vi "main-顶层容器-网络客户端.vi"() -> ()   [LabVIEW 2017]
uses:
  21b310b3-65e2-4238-aede-b4c1b8493430.vi
panel:
  out "错误输出":errorcluster
  in  "信号-设置":bool=TRUE
  in  "子面板模式":T1
  out "浏览-刷新信号 按钮":refnum<vi>
  out "浏览-停止信号 按钮":refnum<vi>
  out "查询窗口VI-引用":refnum<vi>
  out "管-监测模式状态？":refnum<vi>
  out "管-停止信号（枚举）":refnum<vi>
  out "管-监测窗口 按钮":refnum<vi>
  in  "监-外部停止信号":refnum<vi>
  out "管理窗口VI-引用":refnum<vi>
  out "管-监测窗口VI-控件引用":refnum<vi>
  in  "管理模式":bool
  in  "监测模式":bool
  in  "浏览模式":bool
  in  "设置":bool
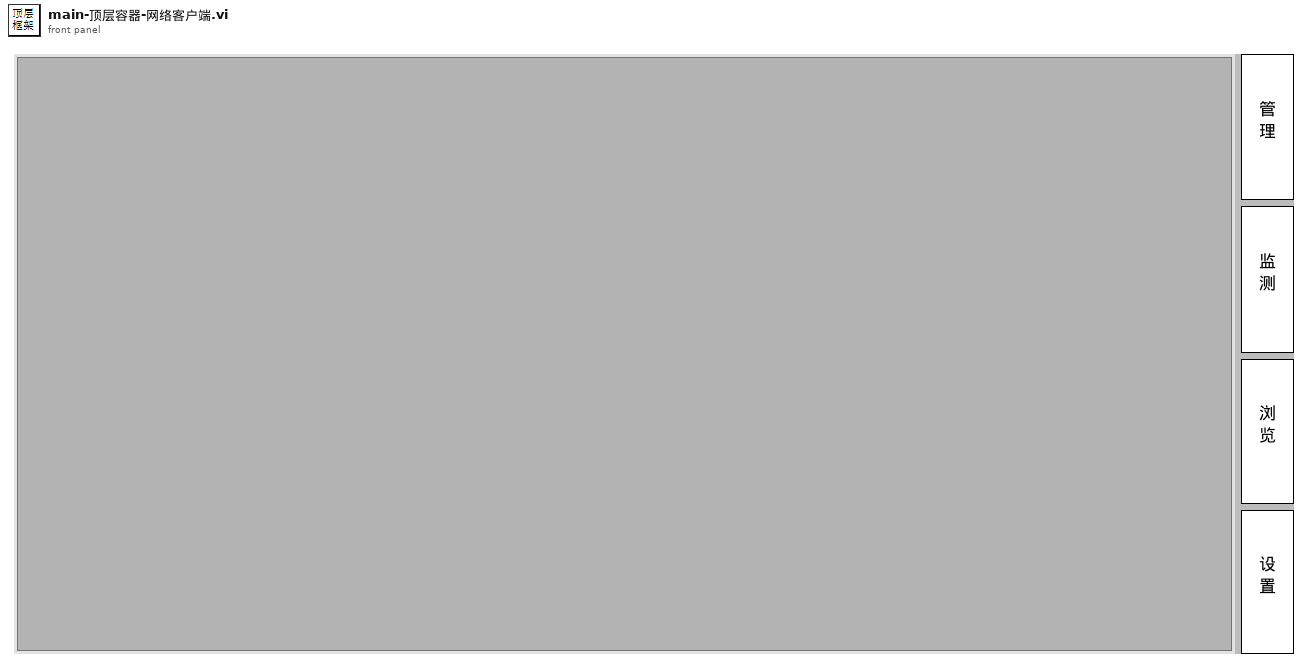
[diagram p1: front panel]
types:
  T1 = typedef "枚举-顶层框架功能模式.ctl" = enum16{"管理模式", "监测模式", "浏览模式"}
  T2 = typedef "簇-输入.ctl" = cluster{"配置文件动作":T3, "数据输入":variant}
  T3 = typedef "枚举-配置文件动作.ctl" = enum16{"初始化加载配置", "读取配置", "写入-屏幕键盘", "写入-静音延迟", "写入-主要探头类型", "写入-串口配置", "写入-累积定时", "写入-导出定时", "保存配置到文件"}
  T4 = enum8{"Enabled", "Disabled", "Disabled and Grayed Out"}
  T5 = typedef "簇-配置文件内容.ctl" = cluster{"调试模式？":bool, "屏幕键盘？":bool, "软件版本":string, "静音延迟 s":u16, "主要探头类型":T6, "串口配置":cluster{"COM口":refnum<visa-resource-name>, "波特率":enum16{"9600", "19200"}, "读写超时ms":i16, "丢包判定次数":i16}, "定时配置-累积分段":T7, "定时配置-自动导出":cluster{"定时配置-自动导出":T7, "分别导出?":bool}}
  T6 = typedef "枚举-主要探头类型.ctl" = enum16{"网络探头", "串口探头"}
  T7 = typedef "簇-定时配置.ctl" = cluster{"定时模式":enum16{"绝对时间", "相对时间"}, "单位":enum16{"年", "月", "日", "时", "分"}, "间隔":u8, "目标时刻":timestamp}
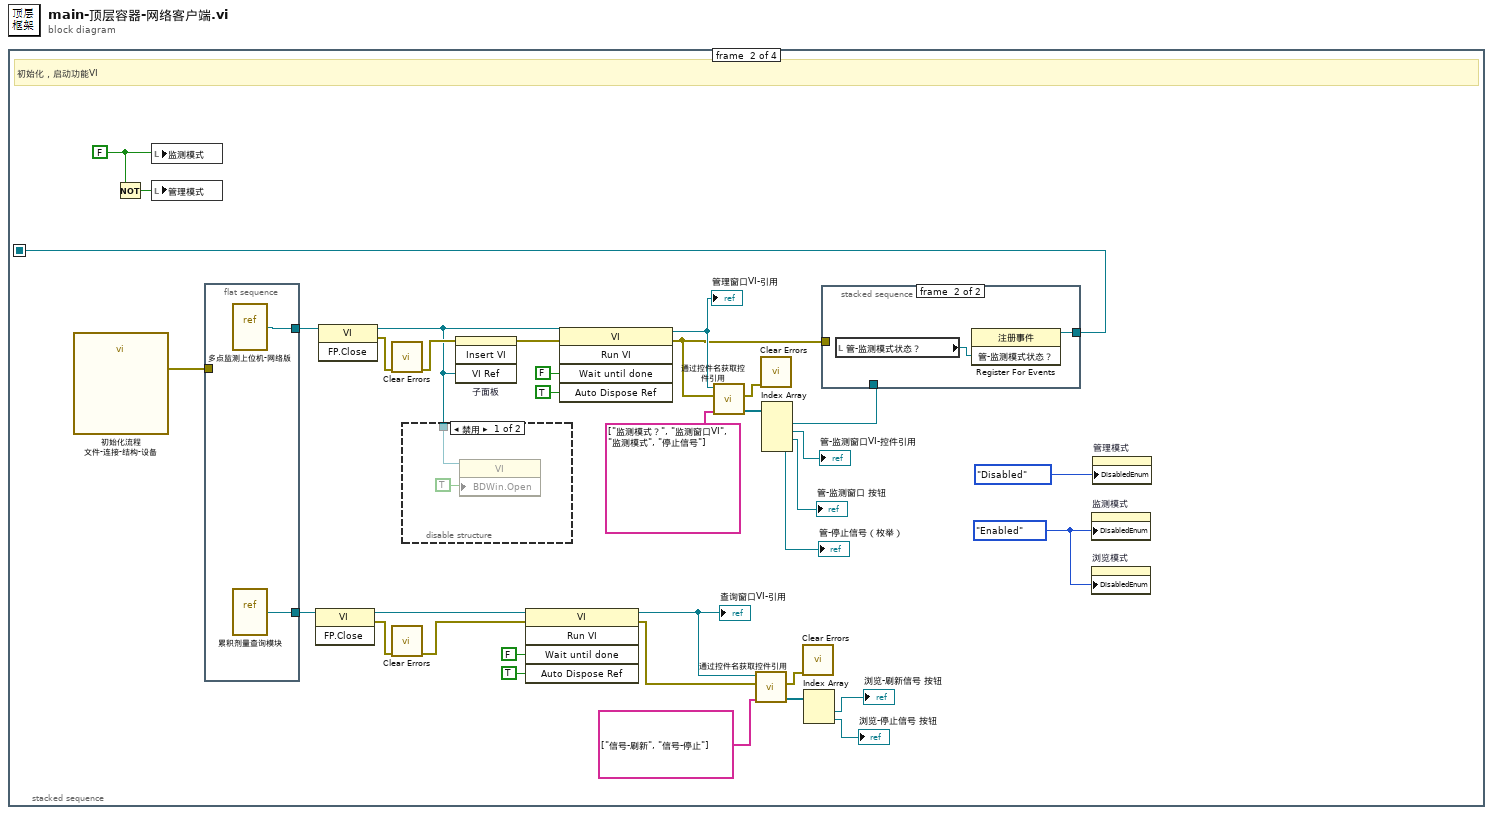
[diagram p0: block diagram]
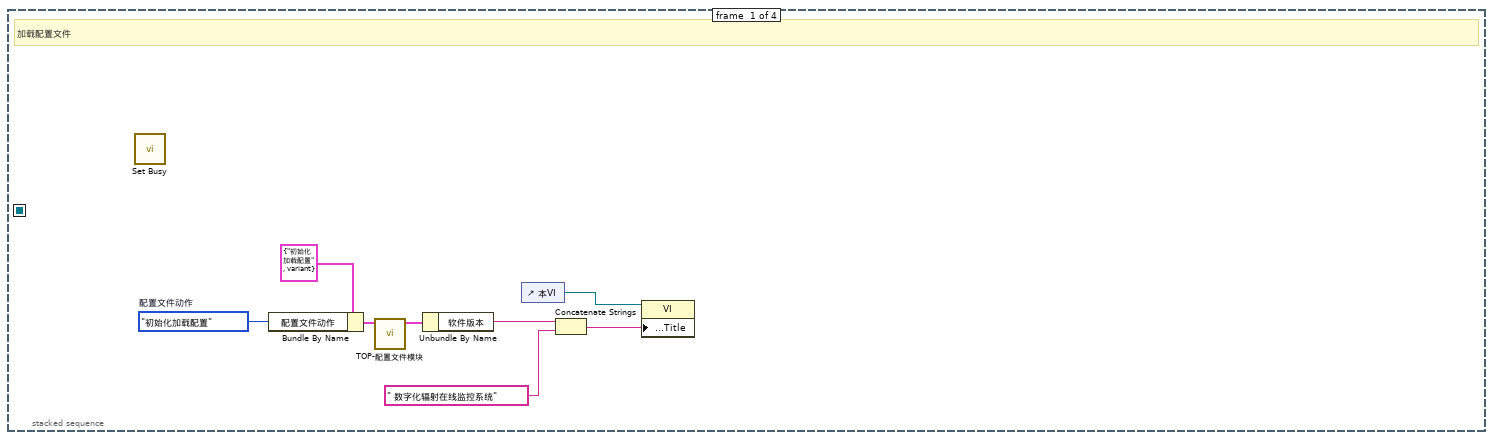
[diagram p2: hidden frame]
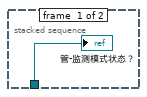
[diagram p4: hidden frame]
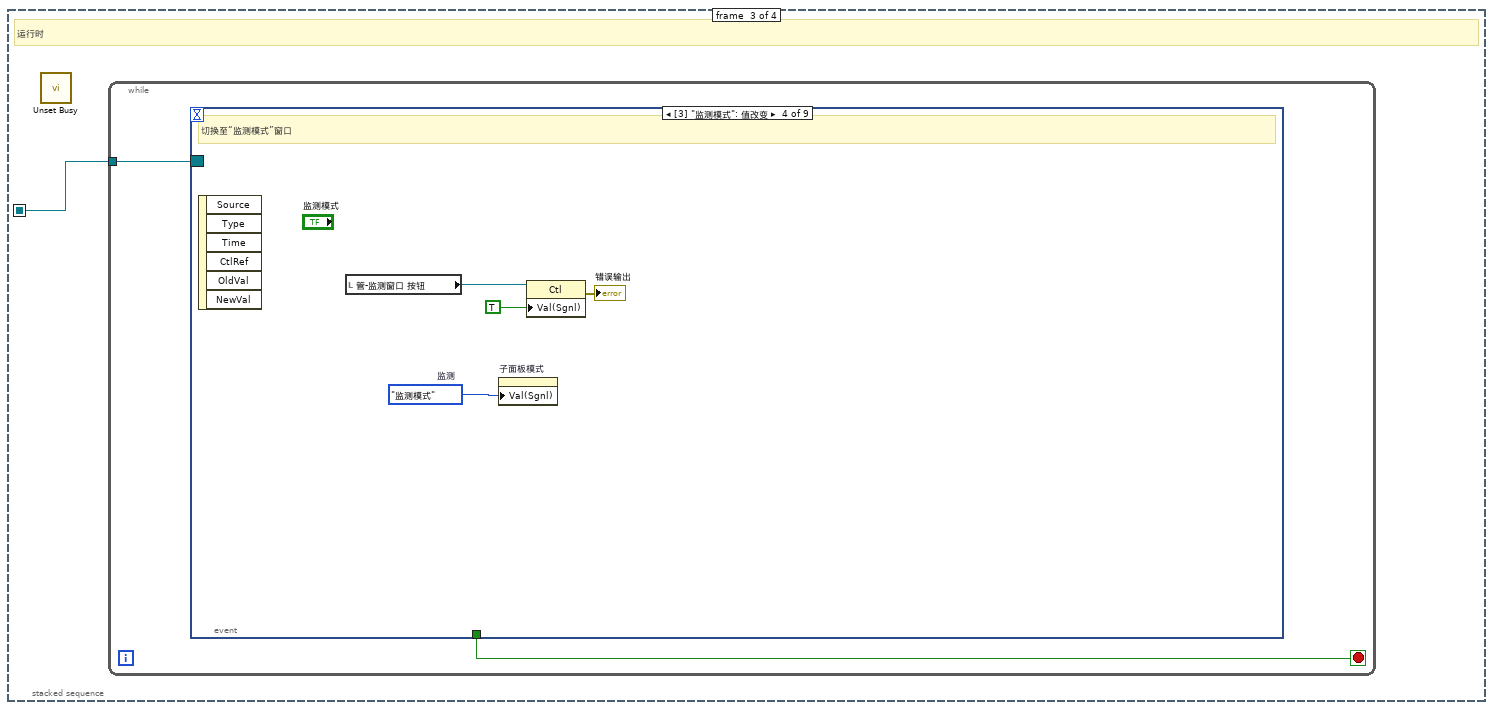
[diagram p5: hidden frame]
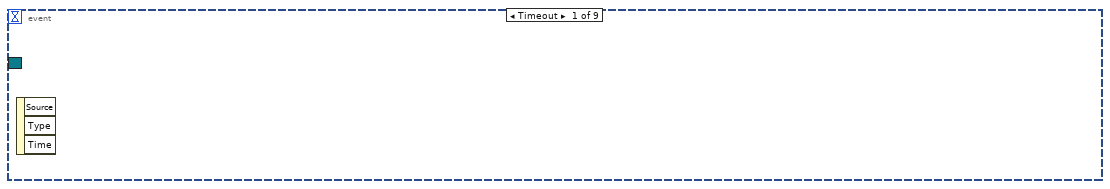
[diagram p6: hidden frame]
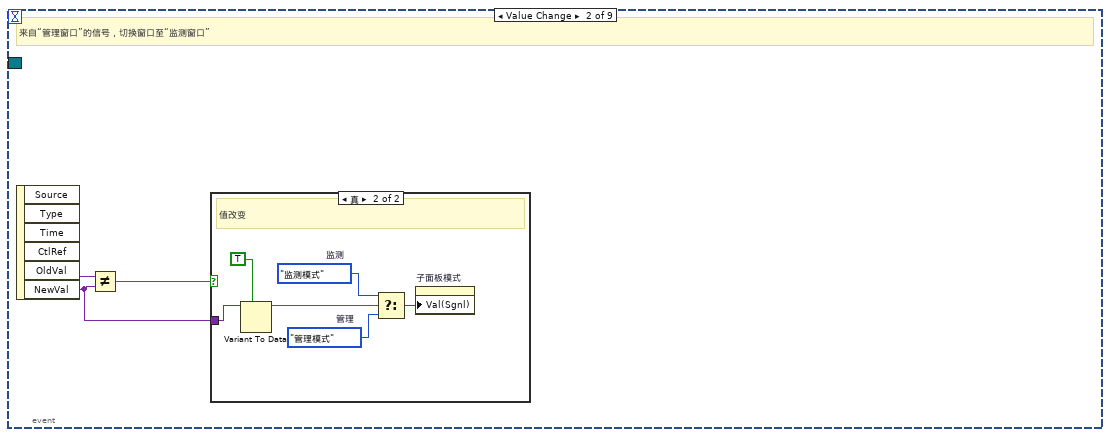
[diagram p7: hidden frame]
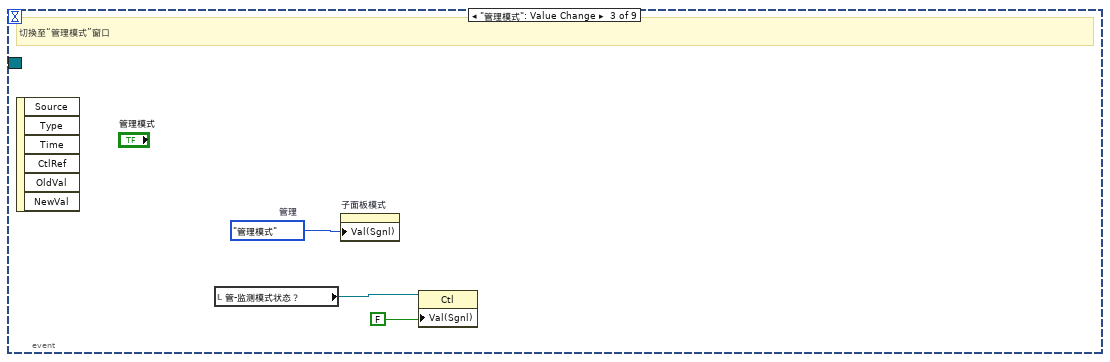
[diagram p9: hidden frame]
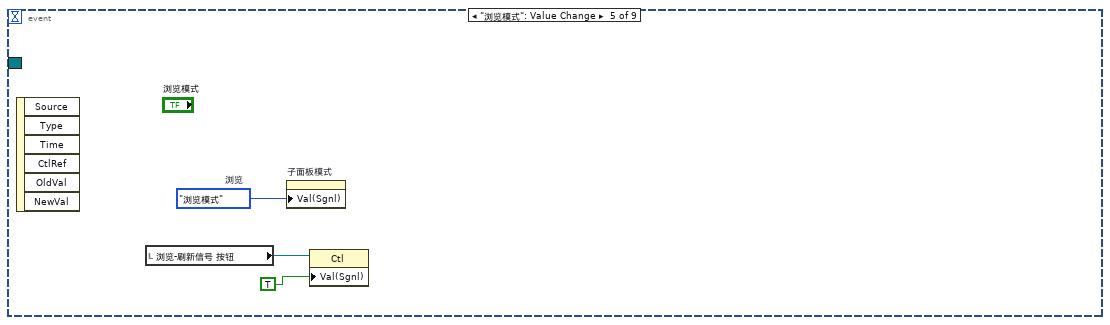
[diagram p10: hidden frame]
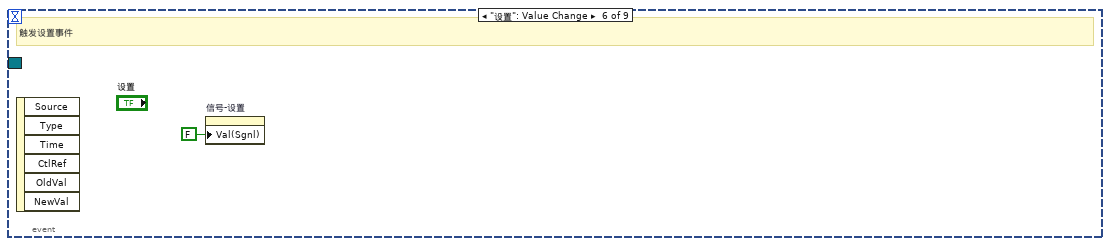
[diagram p11: hidden frame]
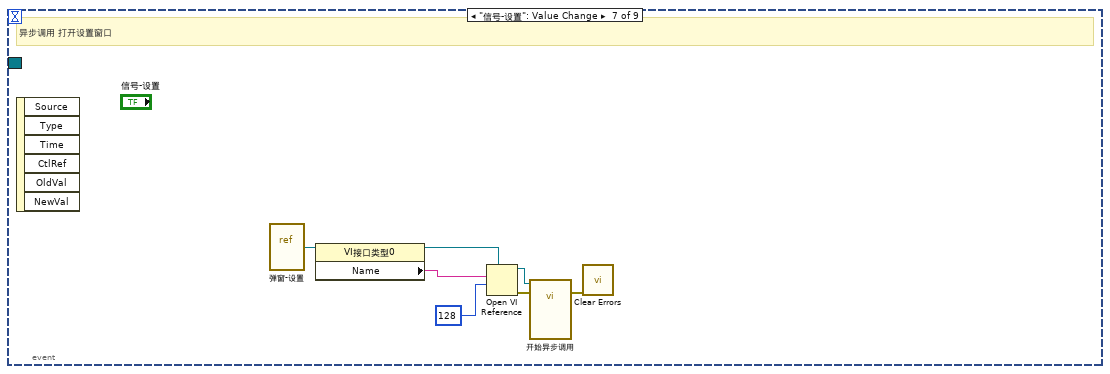
[diagram p12: hidden frame]
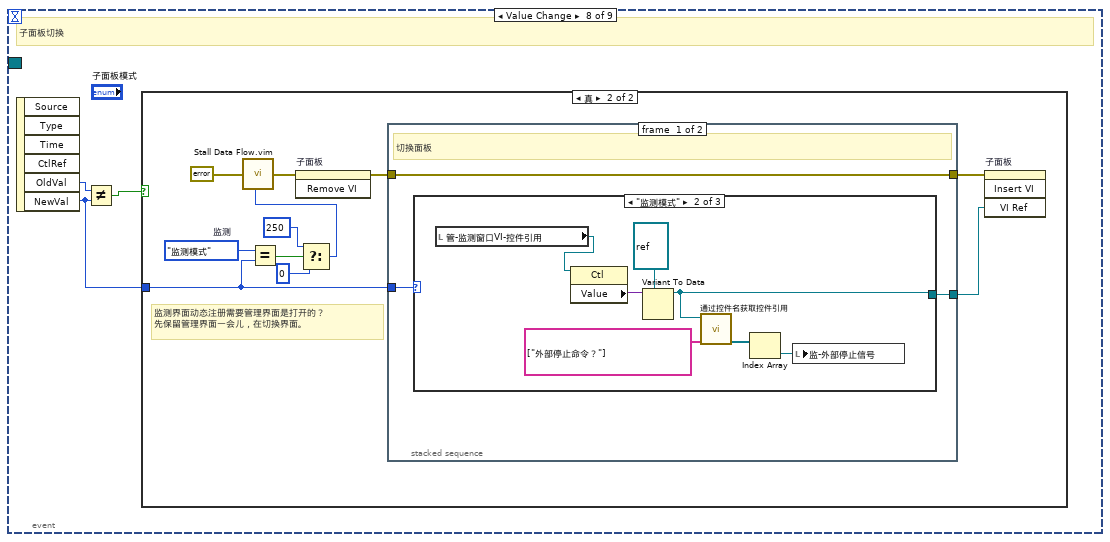
[diagram p13: hidden frame]
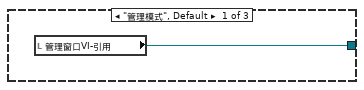
[diagram p15: hidden frame]
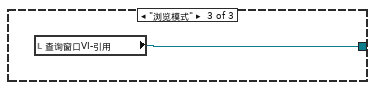
[diagram p16: hidden frame]
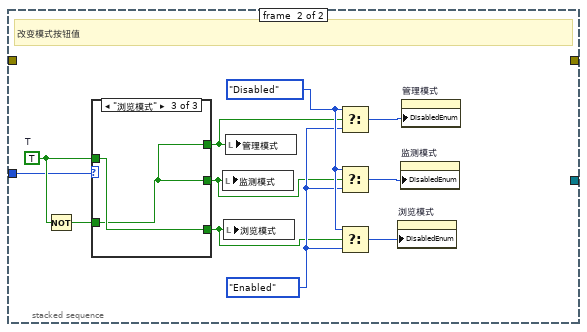
[diagram p17: hidden frame]
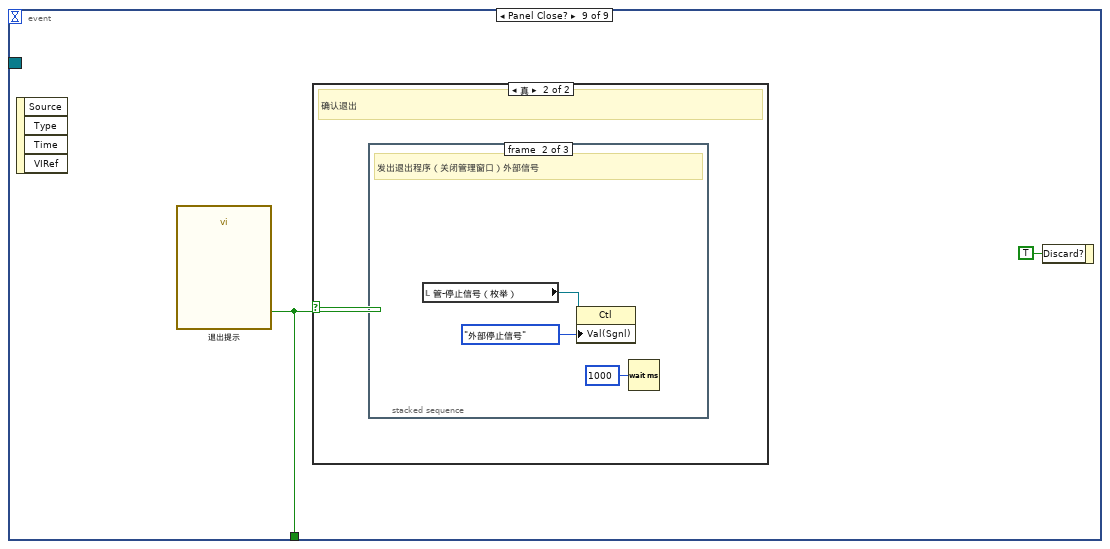
[diagram p20: hidden frame]
diagram:
  n1 = stacked-sequence {
    seq-local: [_ w36 _ _] -> [_ _ w51 _]
    frame #0 {
      w6 = 枚举-配置文件动作."初始化加载配置"  # 配置文件动作
      # "加载配置文件"
      n2 = call <vilib>:"Set Busy.vi"() -> ()  [unwired: 10 in, 2 out]
      n3 = Bundle By Name(cluster=T2 {"配置文件动作"=enum."初始化加载配置", "数据输入"=variant} ("输入"), "配置文件动作"=w6) -> (w7:T2)
      n4 = call "TOP-配置文件模块.vi"("输入"=w7) -> ("配置文件"=w5:T5)  [unwired: 9 in, 1 out]
      n5 = Unbundle By Name(w5) -> ("软件版本"=w1:string)
      n6 = control-ref of="本VI"() -> (w4:refnum<vi>)
      n7 = Concatenate Strings(w1, " 数字化辐射在线监控系统" ("前面板窗口:标题")) -> (w3:string)
      n8 = property class="VI"(reference=w4, "Front Panel.Title"=w3) -> ()  [unwired: 1 in, 2 out]
    }
    frame #1 {
      w9 = T4."Enabled" ("禁用")
      w43 = FALSE ("监测模式")
      # "初始化，启动功能VI"
      n9 = call "初始化流程 文件-连接-结构-设备.vi"() -> ("error out"=w23:errorcluster)  [unwired: 10 in, 1 out]
      n10 = Not(x=w43) -> (.not. x?=w42:bool)
      n11 = local write "监测模式"(w43) -> ()
      n12 = local write "管理模式"(w42) -> ()
      n13 = flat-sequence {
        tunnel: [w45] -> w31
        tunnel: w23 -> [_]
        tunnel: [w44] -> w21
        frame #0 {
          n14 = vi-ref "多点监测上位机-网络版.vi"() -> (w45:refnum<vi>)
          n15 = vi-ref "累积剂量查询模块.vi"() -> (w44:refnum<vi>)
        }
      }
      n16 = invoke class="VI" method="FP.Close"(reference=w21) -> (reference out=w18:refnum<vi>, error out=w22:errorcluster)  [unwired: 2 in, 1 out]
      n17 = invoke class="VI" method="FP.Close"(reference=w31) -> (reference out=w27:refnum<vi>, error out=w29:errorcluster)  [unwired: 2 in, 1 out]
      n18 = call <vilib>:"Clear Errors.vi"("error in (no error)"=w29) -> ("error out"=w28:errorcluster)  [unwired: 5 in, 1 out]
      n19 = call <vilib>:"Clear Errors.vi"("error in (no error)"=w22) -> ("error out"=w17:errorcluster)  [unwired: 5 in, 1 out]
      n20 = disable-structure shown="禁用" {
        disable-tunnel: w27 -> [w47 _]
        frame Disabled {
          n21 = property class="VI"(reference=w47, "BDWin.Open"=TRUE ("程序框图窗口:打开")) -> ()  [unwired: 1 in, 2 out]
        }
        frame Enabled {
        }
      }
      n22 = invoke on="子面板" class="子面板" method="Insert VI"(error in=w28, "VI Ref"=w27) -> (error out=w25:errorcluster)  [unwired: 2 in, 3 out]
      n23 = invoke class="VI" method="Run VI"(reference=w18, error in=w17, "Wait until done"=FALSE ("结束前等待"), "Auto Dispose Ref"=TRUE ("自动销毁引用")) -> (reference out=w13:refnum<vi>, error out=w12:errorcluster)  [unwired: 1 in, 3 out]
      "查询窗口VI-引用" <- w13
      n24 = invoke class="VI" method="Run VI"(reference=w27, error in=w25, "Wait until done"=FALSE ("结束前等待"), "Auto Dispose Ref"=TRUE ("自动销毁引用")) -> (reference out=w37:refnum<vi>, error out=w26:errorcluster)  [unwired: 1 in, 3 out]
      "管理窗口VI-引用" <- w37
      n25 = call "通过控件名获取控件引用.vi"("控件名数组"=string[] ["监测模式？", "监测窗口VI", "监测模式", "停止信号"], "错误输入（无错误）"=w26, "VI引用"=w37) -> ("控件引用输出"=w39:refnum<vi>[], "错误输出"=w30:errorcluster)  [unwired: 6 in, 1 out]
      n26 = call "通过控件名获取控件引用.vi"("控件名数组"=string[] ["信号-刷新", "信号-停止"], "错误输入（无错误）"=w12, "VI引用"=w13) -> ("控件引用输出"=w15:refnum<vi>[], "错误输出"=w16:errorcluster)  [unwired: 6 in, 1 out]
      n27 = call <vilib>:"Clear Errors.vi"("error in (no error)"=w30) -> ()  [unwired: 5 in, 2 out]
      n28 = Index Array(array=w39) -> (element #1=w24:refnum<vi>, element #2=→"管-监测窗口VI-控件引用":refnum<vi>, element #3=→"管-监测窗口 按钮":refnum<vi>, element #4=→"管-停止信号（枚举）":refnum<vi>)  [unwired: 4 in]
      n29 = call <vilib>:"Clear Errors.vi"("error in (no error)"=w16) -> ()  [unwired: 5 in, 2 out]
      n30 = Index Array(array=w15) -> (element #1=→"浏览-刷新信号 按钮":refnum<vi>, element #2=→"浏览-停止信号 按钮":refnum<vi>)  [unwired: 2 in]
      n31 = stacked-sequence {
        tunnel: [_ w50] -> w36
        tunnel: w26 -> [_ _]
        tunnel: w24 -> [w48 _]
        frame #0 {
          "管-监测模式状态？" <- w48
        }
        frame #1 {
          n32 = local read "管-监测模式状态？"() -> (w49:refnum<vi>)
          n33 = register-events(w49) -> (reference out=w50:refnum<event-registration>)  [unwired: 2 in, 1 out]
        }
      }
      n34 = property on="监测模式" class="Bool (严格)"("DisabledEnum"=w9) -> ()  [unwired: 2 in, 2 out]
      n35 = property on="浏览模式" class="Bool (严格)"("DisabledEnum"=w9) -> ()  [unwired: 2 in, 2 out]
      n36 = property on="管理模式" class="Bool (严格)"("DisabledEnum"=T4."Disabled" ("禁用")) -> ()  [unwired: 2 in, 2 out]
    }
    frame #2 {
      # "运行时"
      n37 = call <vilib>:"Unset Busy.vi"() -> ()  [unwired: 11 in, 1 out]
      n38 = while {
        tunnel: w51 -> [w52]
        stop <- w53 stop-if-true
        n39 = event shown="[3] \"监测模式\": 值改变" {
          selector: w52 -> [_ _ _ _ _ _ _ _ _]
          dyn-events: _ -> [_ _ _ _ _ _ _ _ _]
          timeout: _ -> [_ _ _ _ _ _ _ _ _]
          tunnel: [_ _ _ _ _ _ _ _ w124] -> w53
          event Timeout {
            n40 = event-data() -> ()  [unwired: 1 in, 3 out]
          }
          event Value Change {
            # "来自“管理窗口”的信号，切换窗口至“监测窗口”"
            n41 = event-data() -> ("OldVal"=w56:variant, "NewVal"=w55:variant)  [unwired: 1 in, 4 out]
            n42 = Not Equal?(x=w56, y=w55) -> (x != y?=w54:bool)
            n43 = case shown="真" w54 {
              tunnel: w55 -> [_ w59]
              frame False {
              }
              frame True {
                w60 = 枚举-顶层框架功能模式."管理模式"  # 管理
                w58 = 枚举-顶层框架功能模式."监测模式"  # 监测
                # "值改变"
                n44 = Variant To Data(type=TRUE, Variant=w59) -> (data=w61:bool)  [unwired: 1 in, 1 out]
                n45 = Select(t=w58, s=w61, f=w60) -> (s? t:f=w57:T1)
                n46 = property on="子面板模式" class="Enum (严格)"("Val(Sgnl)"=w57) -> ()  [unwired: 2 in, 2 out]
              }
            }
          }
          event "管理模式": Value Change {
            w63 = 枚举-顶层框架功能模式."管理模式"  # 管理
            # "切换至“管理模式”窗口"
            n47 = event-data() -> ()  [unwired: 1 in, 6 out]
            n48 = local read "管-监测模式状态？"() -> (w64:refnum<vi>)
            n49 = property on="子面板模式" class="Enum (严格)"("Val(Sgnl)"=w63) -> ()  [unwired: 2 in, 2 out]
            n50 = property class="Ctl"(reference=w64, "Val(Sgnl)"=FALSE ("管理模式")) -> ()  [unwired: 1 in, 2 out]
          }
          event "监测模式": Value Change {
            w67 = 枚举-顶层框架功能模式."监测模式"  # 监测
            # "切换至“监测模式”窗口"
            n51 = event-data() -> ()  [unwired: 1 in, 6 out]
            n52 = local read "管-监测窗口 按钮"() -> (w69:refnum<vi>)
            n53 = property on="子面板模式" class="Enum (严格)"("Val(Sgnl)"=w67) -> ()  [unwired: 2 in, 2 out]
            n54 = property class="Ctl"(reference=w69, "Val(Sgnl)"=TRUE ("监测模式")) -> (error out=→"错误输出":errorcluster)  [unwired: 1 in, 1 out]
          }
          event "浏览模式": Value Change {
            w72 = 枚举-顶层框架功能模式."浏览模式"  # 浏览
            n55 = event-data() -> ()  [unwired: 1 in, 6 out]
            n56 = local read "浏览-刷新信号 按钮"() -> (w71:refnum<vi>)
            n57 = property on="子面板模式" class="Enum (严格)"("Val(Sgnl)"=w72) -> ()  [unwired: 2 in, 2 out]
            n58 = property class="Ctl"(reference=w71, "Val(Sgnl)"=TRUE) -> ()  [unwired: 1 in, 2 out]
          }
          event "设置": Value Change {
            # "触发设置事件"
            n59 = event-data() -> ()  [unwired: 1 in, 6 out]
            n60 = property on="信号-设置" class="Bool (严格)"("Val(Sgnl)"=FALSE ("值(信号)")) -> ()  [unwired: 2 in, 2 out]
          }
          event "信号-设置": Value Change {
            # "异步调用 打开设置窗口"
            n61 = event-data() -> ()  [unwired: 1 in, 6 out]
            n62 = vi-ref "弹窗-设置.vi"() -> (w80:refnum<vi>)
            n63 = property class="VI接口类型0"(reference=w80) -> (reference out=w74:refnum<vi>, "Name"=w79:string)  [unwired: 1 in, 1 out]
            n64 = Open VI Reference(type specifier VI Refnum (for type only)=w74, vi path=w79, options=128 ("选项")) -> (vi reference=w77:refnum<vi>, error out=w76:errorcluster)  [unwired: 3 in]
            n65 = call-by-ref "开始异步调用"(reference=w77, error in=w76) -> (error out=w75:errorcluster)  [unwired: 12 in, 1 out]
            n66 = call <vilib>:"Clear Errors.vi"("error in (no error)"=w75) -> ()  [unwired: 5 in, 2 out]
          }
          event Value Change {
            # "子面板切换"
            n67 = event-data() -> ("OldVal"=w83:T1, "NewVal"=w81:T1)  [unwired: 1 in, 4 out]
            n68 = Not Equal?(x=w83, y=w81) -> (x != y?=w82:bool)
            n69 = case shown="真" w82 {
              tunnel: w81 -> [_ w89]
              frame False {
              }
              frame True {
                w88 = 枚举-顶层框架功能模式."监测模式"  # 监测
                # "监测界面动态注册需要管理界面是打开的？\n先保留管理界面一会儿，在切换界面。"
                n70 = Equal?(x=w88, y=w89) -> (x = y?=w87:bool)
                n71 = Select(t=u32 250 ("milliseconds to wait"), s=w87, f=u32 0 ("milliseconds to wait")) -> (s? t:f=w84:u32)
                n72 = call "Stall Data Flow.vim"("value in"=errorcluster {"status"=FALSE, "code"=0, "source"=""} ("错误输入（无错误）"), "milliseconds to wait"=w84) -> ("value out"=w90:errorcluster)  [unwired: 1 out]
                n73 = invoke on="子面板" class="子面板" method="Remove VI"(error in=w90) -> (error out=w94:errorcluster)  [unwired: 2 in, 2 out]
                n74 = stacked-sequence {
                  tunnel: w89 -> [w97 w116]
                  tunnel: w94 -> [w96 _]
                  tunnel: [w96 _] -> w93
                  tunnel: [w95 _] -> w92
                  frame #0 {
                    # "切换面板"
                    n75 = case shown="\"监测模式\"" w97 {
                      tunnel: [w98 w99 w106] -> w95
                      frame "管理模式", Default {
                        n76 = local read "管理窗口VI-引用"() -> (w98:refnum<vi>)
                      }
                      frame "监测模式" {
                        n77 = local read "管-监测窗口VI-控件引用"() -> (w100:refnum<vi>)
                        n78 = property class="Ctl"(reference=w100) -> ("Value"=w101:variant)  [unwired: 1 in, 2 out]
                        n79 = Variant To Data(type=refnum<vi> refnum ("本VI"), Variant=w101) -> (data=w99:refnum<vi>)  [unwired: 1 in, 1 out]
                        n80 = call "通过控件名获取控件引用.vi"("控件名数组"=string[] ["外部停止命令？"], "VI引用"=w99) -> ("控件引用输出"=w104:refnum<vi>[])  [unwired: 7 in, 2 out]
                        n81 = Index Array(array=w104) -> (element=w105:refnum<vi>)  [unwired: 1 in]
                        n82 = local write "监-外部停止信号"(w105) -> ()
                      }
                      frame "浏览模式" {
                        n83 = local read "查询窗口VI-引用"() -> (w106:refnum<vi>)
                      }
                    }
                  }
                  frame #1 {
                    w114 = T4."Enabled" ("禁用")
                    w115 = T4."Disabled" ("禁用")
                    w117 = TRUE  # T
                    # "改变模式按钮值"
                    n84 = Not(x=w117) -> (.not. x?=w113:bool)
                    n85 = case shown="\"浏览模式\"" w116 {
                      tunnel: w117 -> [w119 w121 w123]
                      tunnel: w113 -> [w118 w120 w122]
                      tunnel: [w119 w120 w122] -> w112
                      tunnel: [w118 w121 w122] -> w111
                      tunnel: [w118 w120 w123] -> w110
                      frame "管理模式", Default {
                      }
                      frame "监测模式" {
                      }
                      frame "浏览模式" {
                      }
                    }
                    n86 = local write "监测模式"(w111) -> ()
                    n87 = local write "浏览模式"(w110) -> ()
                    n88 = local write "管理模式"(w112) -> ()
                    n89 = Select(t=w115, s=w112, f=w114) -> (s? t:f=w107:T4)
                    n90 = Select(t=w115, s=w111, f=w114) -> (s? t:f=w108:T4)
                    n91 = Select(t=w115, s=w110, f=w114) -> (s? t:f=w109:T4)
                    n92 = property on="浏览模式" class="Bool (严格)"("DisabledEnum"=w109) -> ()  [unwired: 2 in, 2 out]
                    n93 = property on="监测模式" class="Bool (严格)"("DisabledEnum"=w108) -> ()  [unwired: 2 in, 2 out]
                    n94 = property on="管理模式" class="Bool (严格)"("DisabledEnum"=w107) -> ()  [unwired: 2 in, 2 out]
                  }
                }
                n95 = invoke on="子面板" class="子面板" method="Insert VI"(error in=w93, "VI Ref"=w92) -> ()  [unwired: 2 in, 4 out]
              }
            }
          }
          event Panel Close? {
            n96 = event-data() -> ()  [unwired: 1 in, 4 out]
            n97 = call "退出提示"() -> ("确定"=w124:bool)  [unwired: 10 in, 1 out]
            n98 = case shown="真" w124 {
              frame False {
                # "取消推出"
              }
              frame True {
                # "确认退出"
                n99 = stacked-sequence {
                  frame #0 {
                    w126 = TRUE ("监测模式")
                    # "判断是否“监测模式”，是的话先退出监测模式"
                    n100 = local read "浏览-停止信号 按钮"() -> (w128:refnum<vi>)
                    n101 = property class="Ctl"(reference="监-外部停止信号", "Val(Sgnl)"=w126) -> (error out=w131:errorcluster)  [unwired: 1 in, 1 out]
                    n102 = property class="Ctl"(reference=w128, "Val(Sgnl)"=w126) -> (error out=w127:errorcluster)  [unwired: 1 in, 1 out]
                    n103 = call <vilib>:"Clear Errors.vi"("error in (no error)"=w131) -> ()  [unwired: 5 in, 2 out]
                    n104 = call <vilib>:"Clear Errors.vi"("error in (no error)"=w127) -> ()  [unwired: 5 in, 2 out]
                    n105 = Wait (ms)(milliseconds to wait=u32 1000 ("等待时间（毫秒）")) -> ()  [unwired: 1 out]
                  }
                  frame #1 {
                    # "发出退出程序（关闭管理窗口）外部信号"
                    n106 = local read "管-停止信号（枚举）"() -> (w134:refnum<vi>)
                    n107 = property class="Ctl"(reference=w134, "Val(Sgnl)"=enum16{"内部停止信号", "外部停止信号"}."外部停止信号" ("值(信号)")) -> ()  [unwired: 1 in, 2 out]
                    n108 = Wait (ms)(milliseconds to wait=u32 1000 ("等待时间（毫秒）")) -> ()  [unwired: 1 out]
                  }
                  frame #2 {
                    # "移除"
                    n109 = invoke on="子面板" class="子面板" method="Remove VI"() -> ()  [unwired: 3 in, 3 out]
                  }
                }
              }
            }
            n110 = event-data("Discard?"=TRUE ("放弃？")) -> ()  [unwired: 1 in, 1 out]
          }
        }
      }
    }
    frame #3 {
      # "结束"
      n111 = control-ref of="本VI"() -> (w138:refnum<vi>)
      n112 = invoke class="VI" method="FP.Close"(reference=w138) -> (reference out=w137:refnum<vi>, error out=w136:errorcluster)  [unwired: 2 in, 1 out]
      n113 = invoke class="VI" method="Abort VI"(reference=w137, error in=w136) -> (error out=w135:errorcluster)  [unwired: 1 in, 2 out]
      n114 = call <vilib>:"Clear Errors.vi"("error in (no error)"=w135) -> ()  [unwired: 5 in, 2 out]
    }
  }
